vi "RSquareCalculation.vi"(1 "Extinction ExtinctionUncertainity Size parameter and Number ofS sizes 2":T1={"Extinction"=[], "Extinction Uncertainty"=[], "Size parameters"=[], "Number ofSizes"=0.0, "GeometricCrossSection"=[], "Wave Length"=0.0, "SMPS Sizes"=[], "Concentration"=[], "Double Charge Correction"=FALSE, "Extincation Factor"=1.0, "Diameter Factor"=1.0, "Diameter Offset"=0.0, "Extinction Factor Flag"=FALSE, "Diameter Factor Flag"=FALSE, "Diameter Offset Flag"=FALSE, "Sizes"=[]}, 2 "refractive index, imaginary":sgl=0.1 step=0.01 format="%.3f", 3 "refractive index, real":sgl=1.3 step=0.01 format="%.3f") -> (0 "R-square":dbl)   [LabVIEW 2011]
uses:
  BaesDataTypeDefinition.ctl
  mie2.dll
  <vilib>/Analysis/NI_AALPro.lvlib
panel:
  out "Expected Value For R and I refractive Index":sgl[](array[numeric])
  out "totalscatter 2":sgl
  out "backscatter 2":sgl
  out "<cos(theta)> 3":sgl
  out "extinction 2":sgl
  in  "angles (will compute\n2*angles-1 points from\n0...180 degrees)":u32=2
  # "Mie scattering demo program, August 2005, by Martin Fierz (martin@fierz.ch)\n\nThis VI demonstrates the usage of mie2.dll; a dynamic-link-library which you can call in your LabView program.\nThe demo lets you select the refractive index of a sphere, and the size parameter and computes total scattering,\ntotal extinction and angular distribution of the scattered light for p-, s- and unpolarized light.\nMie2.dll uses the Bohren-Huffman Mie code."
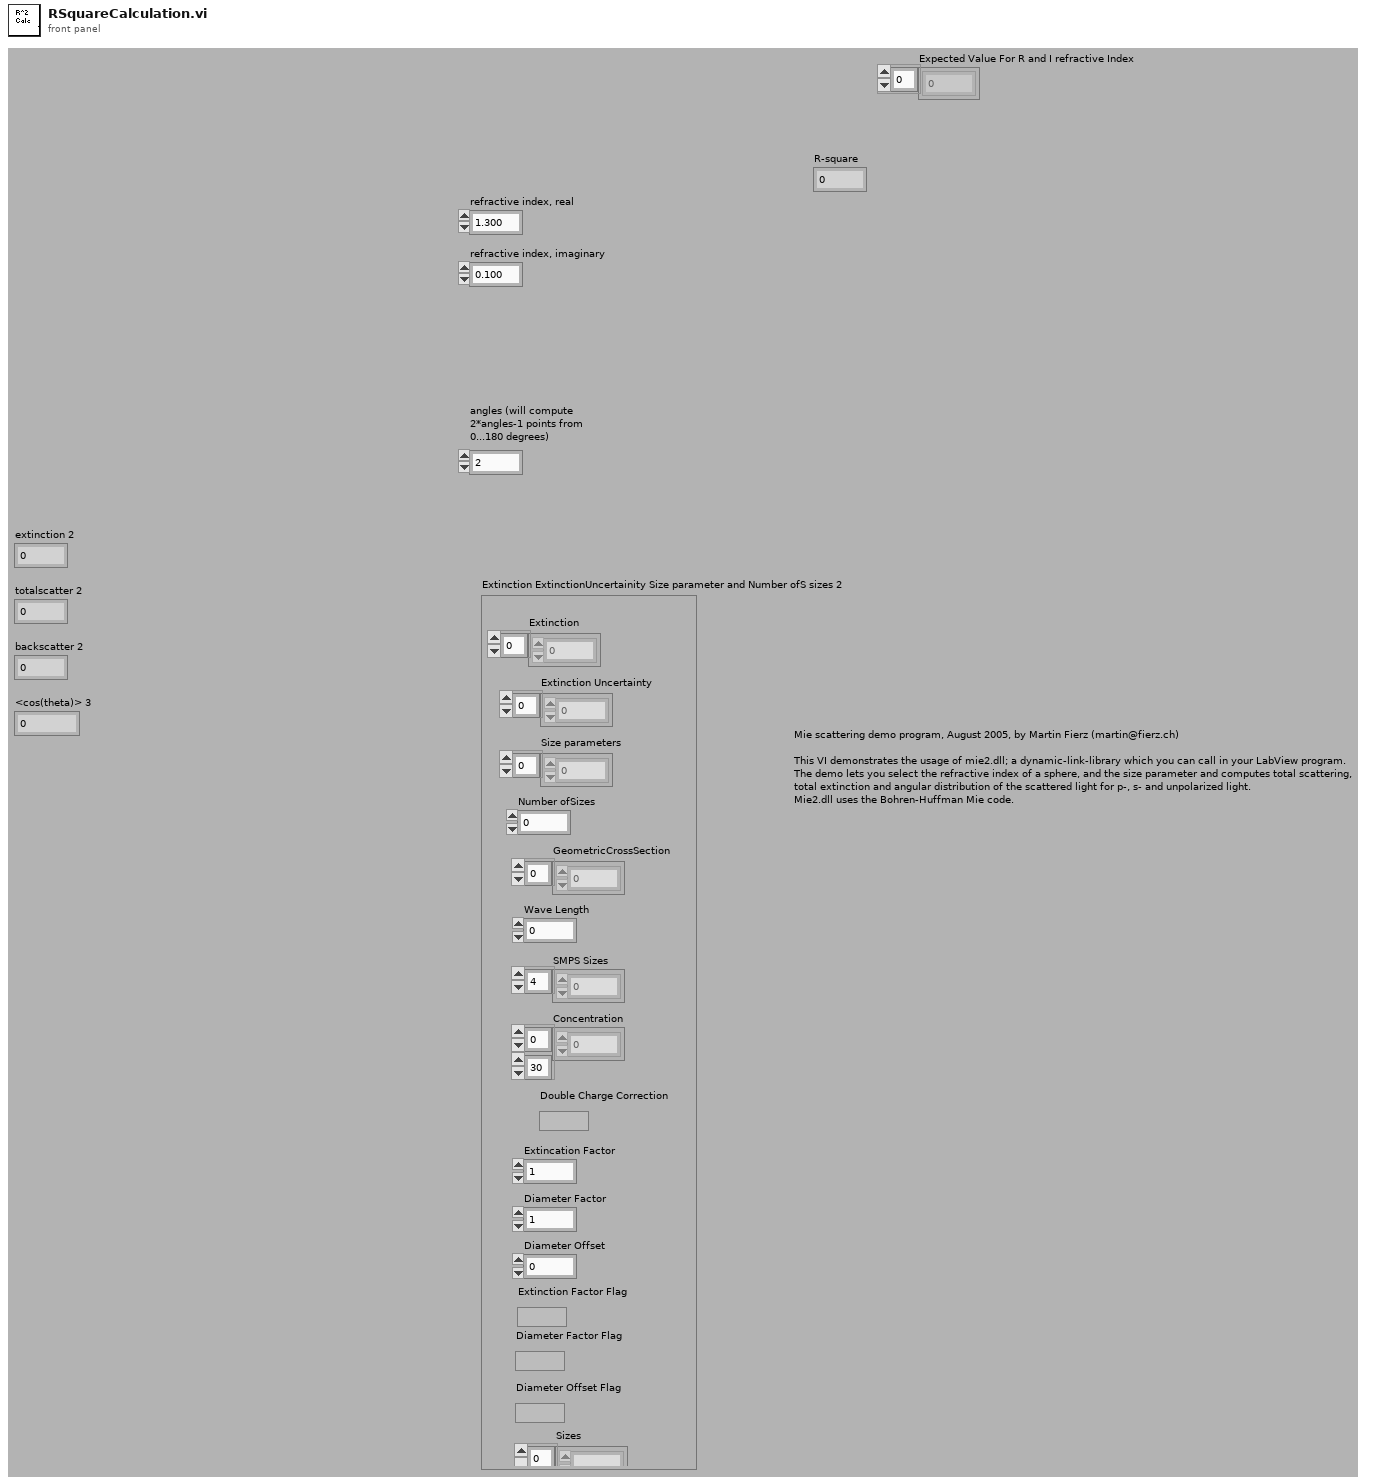
[diagram p1: front panel]
types:
  T1 = typedef "BaesDataTypeDefinition.ctl" = cluster{"Extinction":dbl[], "Extinction Uncertainty":dbl[], "Size parameters":dbl[], "Number ofSizes":dbl, "GeometricCrossSection":dbl[], "Wave Length":dbl, "SMPS Sizes":dbl[], "Concentration":dbl[][], "Double Charge Correction":bool, "Extincation Factor":dbl, "Diameter Factor":dbl, "Diameter Offset":dbl, "Extinction Factor Flag":bool, "Diameter Factor Flag":bool, "Diameter Offset Flag":bool, "Sizes":dbl[]}
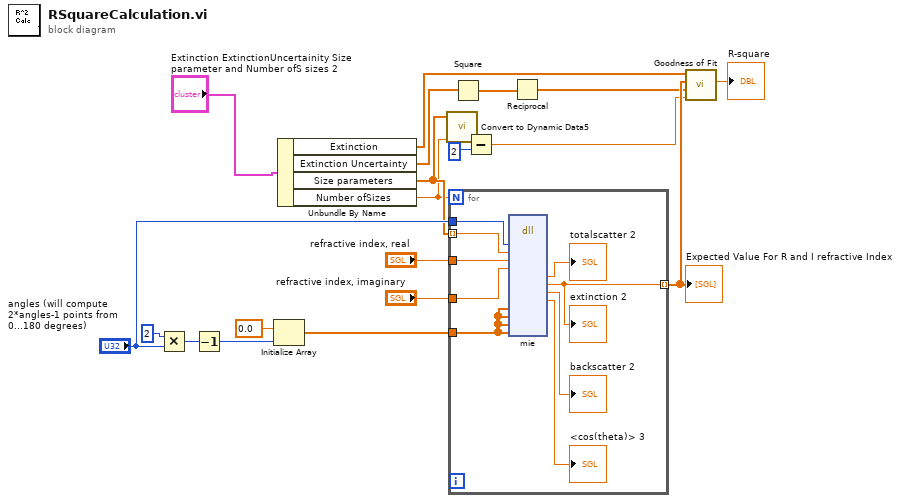
[diagram p0: block diagram]
diagram:
  n1 = Multiply(x=u32 2, y="angles (will compute\n2*angles-1 points from\n0...180 degrees)") -> (x*y=w18:u32)
  n2 = Decrement(x=w18) -> (x-1=w16:u32)
  n3 = Initialize Array(sgl 0.0, w16) -> (w12:sgl[])
  n4 = Unbundle By Name("Extinction ExtinctionUncertainity Size parameter and Number ofS sizes 2") -> ("Extinction"=w4:dbl[], "Extinction Uncertainty"=w3:dbl[], "Size parameters"=w5:dbl[], "Number ofSizes"=w2:dbl)
  n5 = call "Convert to Dynamic Data5"("Array"=w5) -> ()  [unwired: 3 in, 1 out]
  n6 = for {
    N: w2 -> [_]
    tunnel: w12 -> [w26]
    tunnel: "angles (will compute\n2*angles-1 points from\n0...180 degrees)" -> [w25]
    tunnel: "refractive index, real" -> [w24]
    tunnel: "refractive index, imaginary" -> [w23]
    tunnel: w5 -> [w22] mode=indexing
    tunnel: [w20] -> w11 mode=indexing
    n7 = dll-call lib="Z:/Dropbox/Lior Segev/Lior Segev Projects/RI retrieval in Labview/CheckoutCode/mie2.dll" fn="mie"("angles"=w25, "x"=w22, "r"=w24, "i"=w23, "spol_real"=w26, "spol_imaginary"=w26, "ppol_real"=w26, "ppol_imaginary"=w26) -> ("totalscatter"=→"totalscatter 2":sgl, "extinction"=w20:sgl, "backscatter"=→"backscatter 2":sgl, "<cos(theta)>"=→"<cos(theta)> 3":sgl)  [unwired: 16 in, 2 out]
    "extinction 2" <- w20
  }
  "Expected Value For R and I refractive Index" <- w11
  n8 = Square(x=w3) -> (x^2=w10:dbl[])
  n9 = Subtract(x=w2, y=2) -> (x-y=w7:dbl)
  n10 = Reciprocal(x=w10) -> (1/x=w9:dbl[])
  n11 = call <vilib>:"Goodness of Fit.vi"("degree of freedom"=w7, "Weight"=w9, "Best Fit"=w11, "Y"=w4) -> ("R-square"=→"R-square":dbl)  [unwired: 4 in, 3 out]
